vi "Main FPGA 8-axis_2.vi"() -> ()   [LabVIEW 2014]
uses:
  <vilib>/Motion/MotorControl/_s/nism.interpretControlRegister.stateTransition.ctl
  <vilib>/Platform/TimedLoop/XDataNode/timing_clust.ctl
  <vilib>/Platform/TimedLoop/XDataNode/nitl_modes.ctl
  <vilib>/Platform/TimedLoop/XDataNode/wakeup.ctl
  <vilib>/rvi/Emulation/niFpgaGetClockAttributes.vi
  <vilib>/rvi/Emulation/niFpgaSctlEmulationGetInTimedLoop.vi
  <vilib>/rvi/Emulation/niFpgaEmulationReportErrorSimple.vi
  Global FPGA 8-axis.vi
  <vilib>/rvi/eio/common/nirviEmuTemplateMethod_errors.vi
  <vilib>/Motion/MotorControl/_s/nism.interpretControlRegister.indexed.vi
  <vilib>/rvi/Emulation/niFpgaProcessEmulError.vi
  <vilib>/Motion/MotorControl/_s/nism.mdo.read.positionLoopSyncData.vi
  <vilib>/Motion/MotorControl/_s/nism.mdo.read.splineData.vi
  <vilib>/Motion/MotorControl/_s/nism.generateStatusRegister.indexed.vi
  <vilib>/rvi/Emulation/niFpgaCriticalErrorInLSC.vi
  <vilib>/Motion/MotorControl/_s/nism.splineInterpolation.fxp.3.index.vi
  <vilib>/Motion/MotorControl/_s/nism.mdo.handler.indexed.vi
  <vilib>/Motion/SoftMotion/Synchronization/nism.rioScan.generateSyncScan.vi
  <vilib>/eio/EIONode/EIONode.xnode
  <vilib>/Platform/TimedLoop/XDataNode/XDataNode.xnode
  <vilib>/Motion/MotorControl/NI_SoftMotion_MotorControlIP.lvlib
  <vilib>/Platform/TimedLoop/XDataNode/XDNodeRunTimeDep.lvlib
  <vilib>/Motion/SoftMotion/Synchronization/NI_SoftMotion_Synchronization.lvlib
panel:
  in  "Enable Drives?":bool
  out "State":T1=enum."Start --> Initializing" caption="state transition"
  in  "Sync Value":bool
  in  "Sync Enable override?":bool
  in  "Invert direction?":bool
  out "Sync is Fault":bool
  out "Sync is Locked":bool
  in  "minimum pulse":u16=40
  # "Synchronization Loop"
  # "Control Status Loop"
  # "Notes: \n1. This VI provides the communication interface between the NI SoftMotion Engine and the LabVIEW FPGA Module. You must compile this VI for a specific FPGA target before use. After compiling, run the VI before running any of the Express VI examples. For information on moving this example to another FPGA target, refer to ni.com/info and enter info code fpgaex.\n\n2. Only use the Reset Axis button if you are unable to communicate with the axis by any other means. This button resets the device state machine and other VIs to a known state. After resetting the axis, switch the NI Scan Engine from Active Mode to Configuration Mode, then back to Active Mode, before attempting to enable the axis."
  # "(These two buttons \nare for testing\npurposes.)"
  # "Step/Direction Loop"
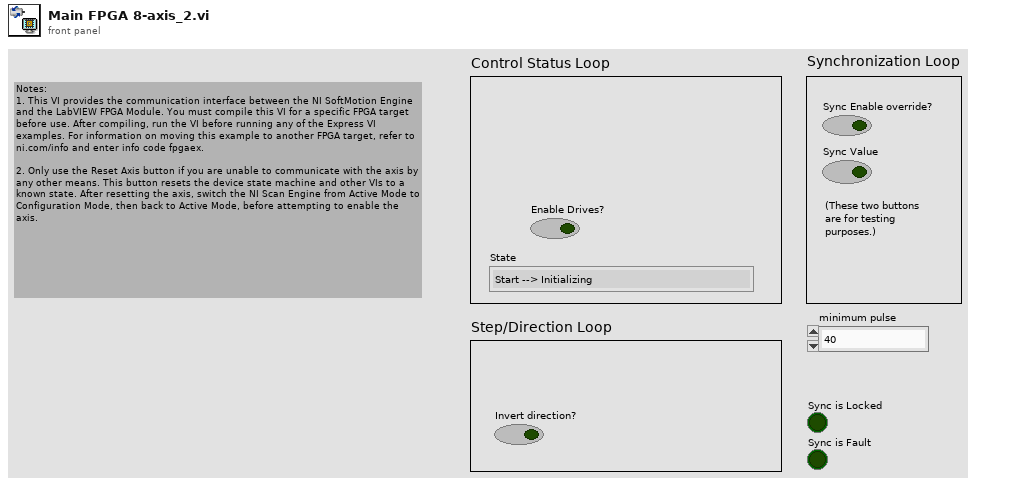
[diagram p1: front panel]
types:
  T1 = typedef "NI_SoftMotion_MotorControlIP.lvlib/nism.interpretControlRegister.stateTransition.ctl" = enum8{"Invalid", "Start --> Initializing", "Initializing --> Disabled", "Disabled --> Ready To Switch On", "Ready To Switch On --> Switched On", "Ready To Switch On --> Disable", "Switched On --> Operation Enable", "Switched On --> Ready To Switch On", "Switched On --> Disabled", "Operation Enable --> Switched On", "Operation Enable --> Ready To Switch On", "Operation Enable --> Disabled", "Fault --> Disabled", "Any --> Fault", "None"}
  T2 = typedef "NI_SoftMotion_MotorControlIP.lvlib/nism.mdo.splineData.ctl" = cluster{"spline type":T3, "traj per/spline per":u16, "spline per/traj per":fxp<+,32,0>}
  T3 = typedef "NI_SoftMotion_MotorControlIP.lvlib/nism.splineInterpolation.type.ctl" = u16
  T4 = typedef "NI_SoftMotion_Synchronization.lvlib/nism.softmotionScan.timerConfig.ctl" = cluster{"target period (clocks)":u16, "host period / target period":u16}
  T5 = typedef "NI_SoftMotion_Synchronization.lvlib/nism.softmotionScan.timerControl.ctl" = cluster{"sm scan":bool, "sm scan count":u32, "sm scan enabled":bool}
  T6 = typedef "XDNodeRunTimeDep.lvlib/timing_clust.ctl" = cluster{"Expected End [f-1]":u64, "Actual End [f-1]":u64, "Finished Late? [f-1]":bool, "Expected End [i-1]":u64, "Actual End [i-1]":u64, "Finished Late? [i-1]":bool, "Expected Start [i]":u64, "Actual Start [i]":u64, "Expected Start [f]":u64, "Actual Start [f]":u64, "Source Name":string, "Structure Name":string, "Period":i64, "Deadline":i64, "Offset":i64, "Start":i64, "Priority":i32, "Timeout":i32, "Mode":T7, "Wakeup Reason":T8, "Error":errorcluster, "Source Type":string, "Secondary Source Type":string, "Global End Time":u64, "Global Start Time":u64, "Frame Duration":u64, "Iteration Duration":u64, "Assigned CPU":i32, "I/O Scan Engine Mode":u32}
  T7 = typedef "XDNodeRunTimeDep.lvlib/nitl_modes.ctl" = enum32{"No Change", "Process missed periods, maintain original phase", "Discard missed periods, maintain original phase", "Process missed periods, ignore original phase", "Discard missed periods, ignore original phase"}
  T8 = typedef "XDNodeRunTimeDep.lvlib/wakeup.ctl" = enum32{"Normal", "Aborted", "Asynchronous wakeup", "Timing source error", "Timed loop error", "Timeout"}
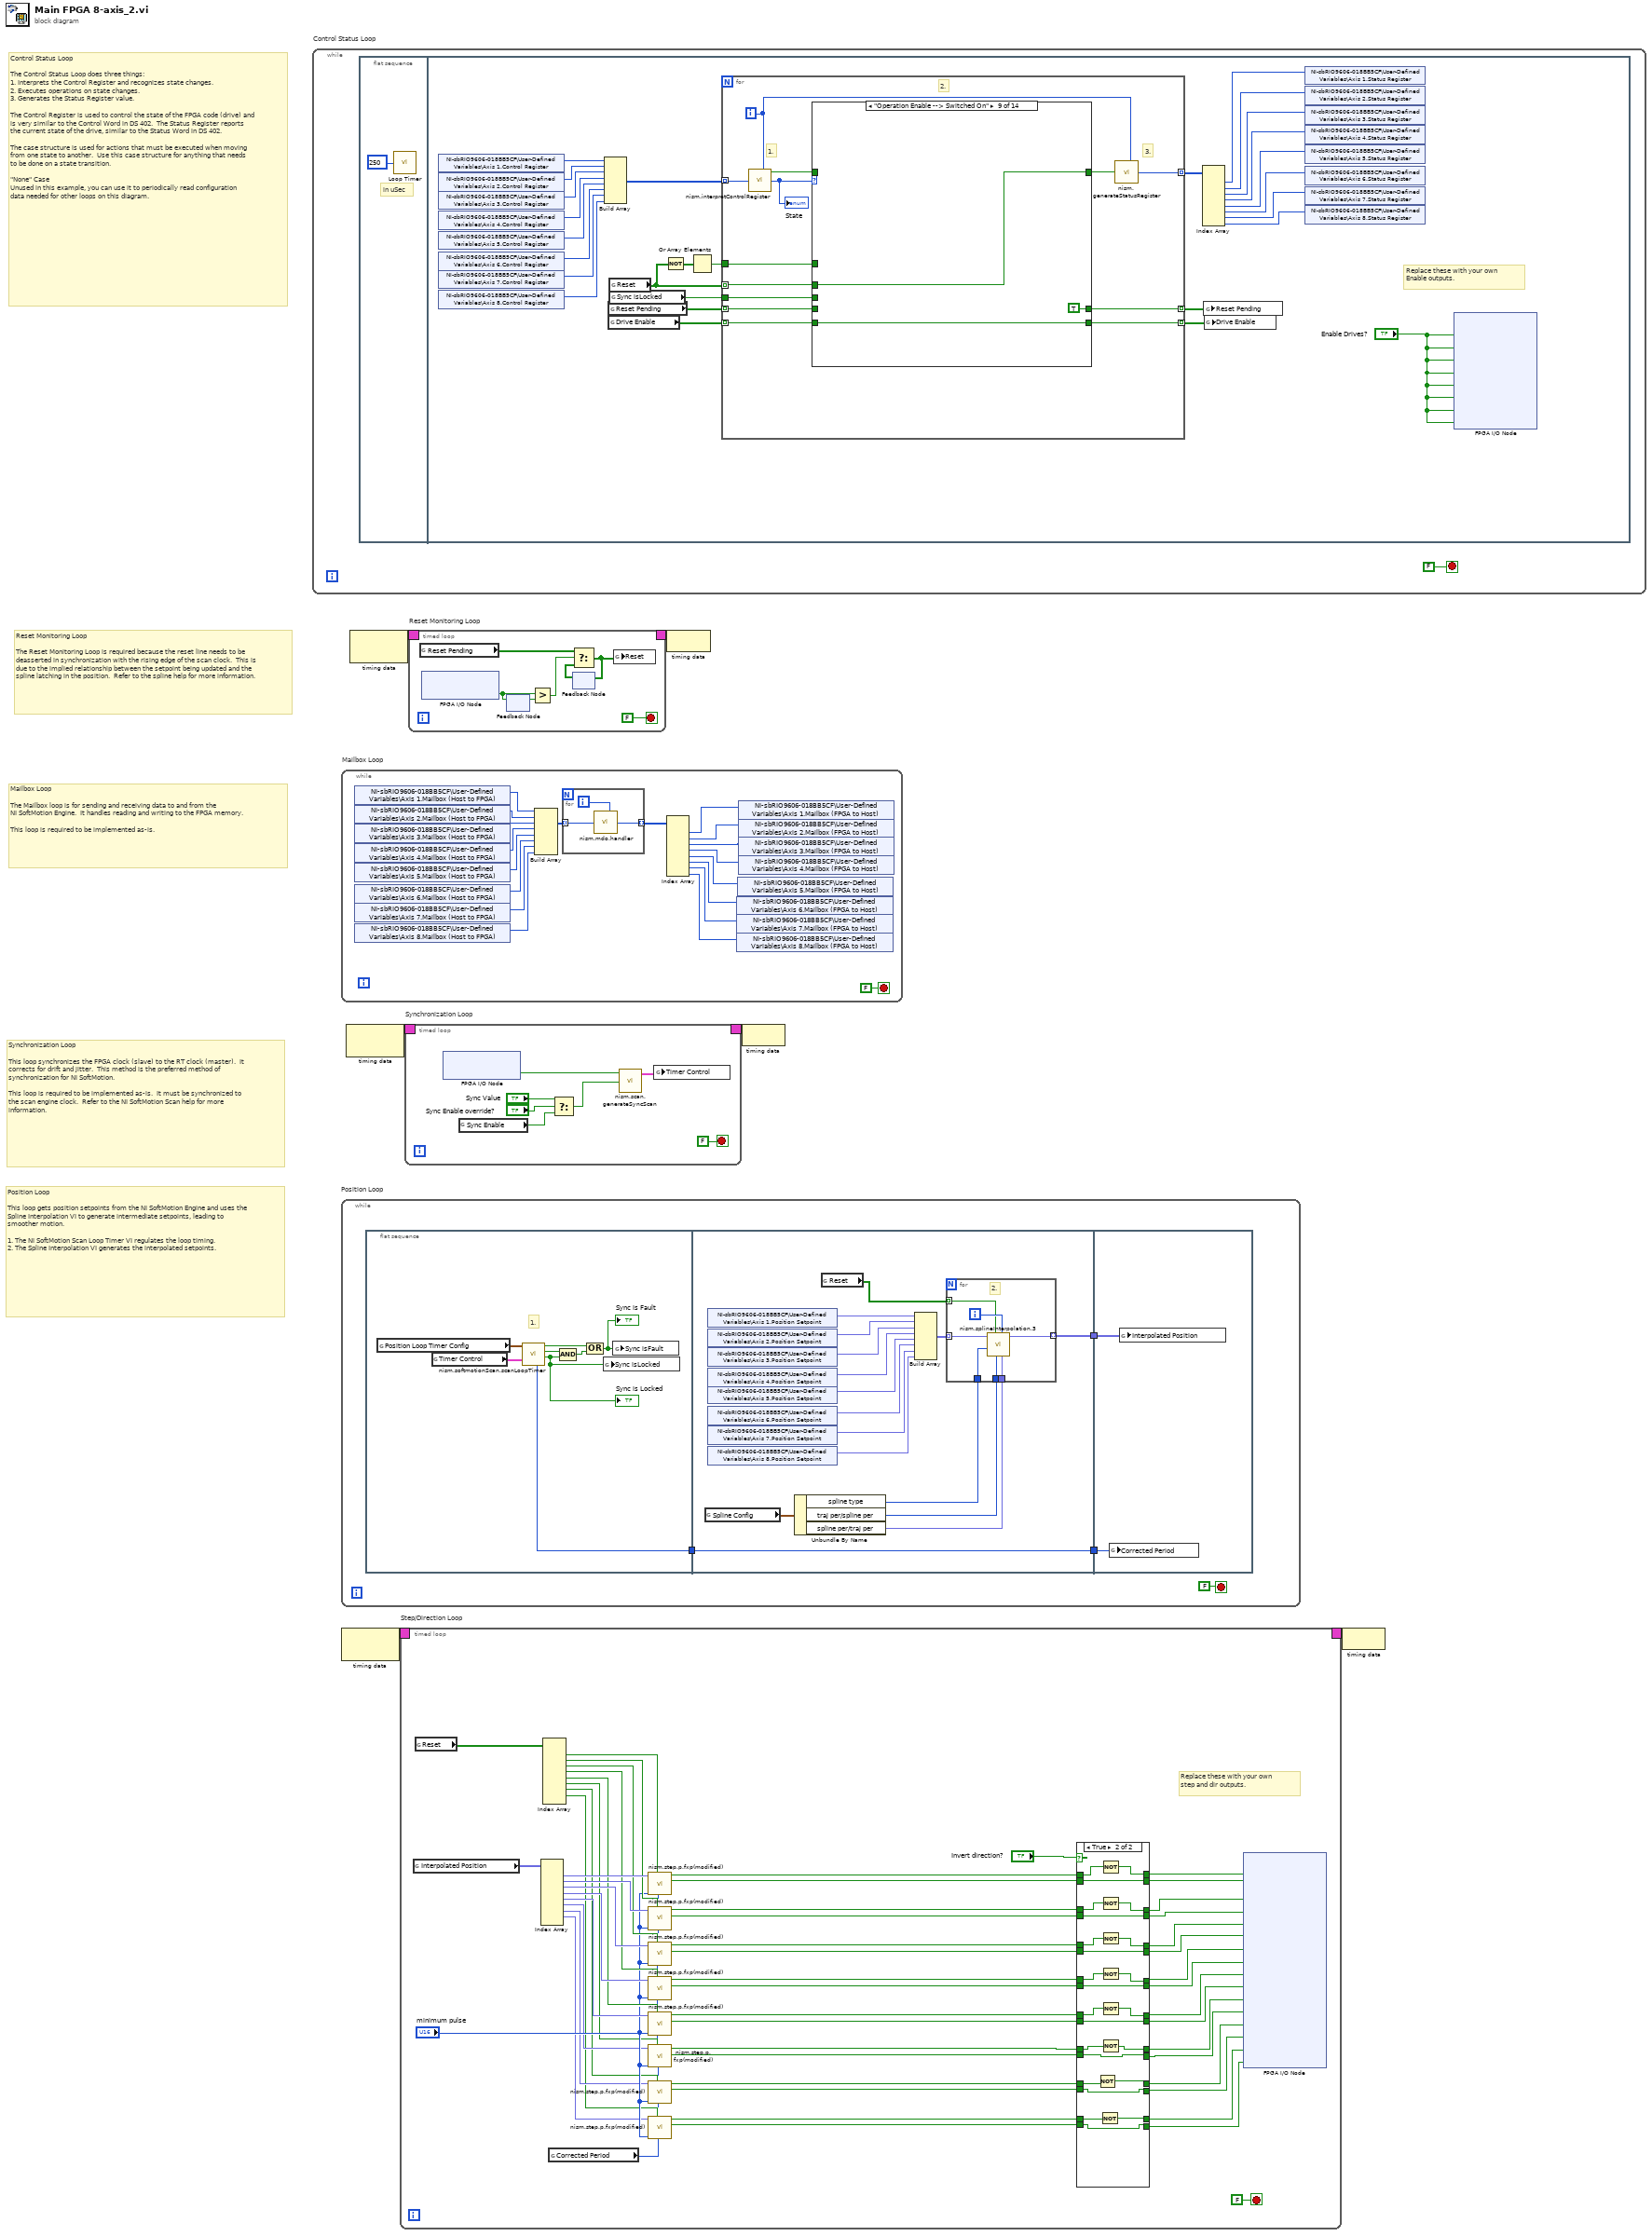
[diagram p0: block diagram]
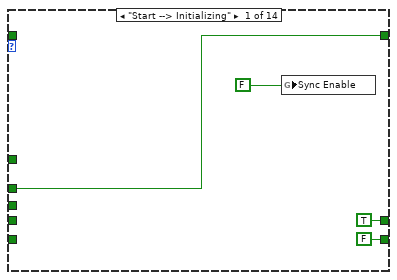
[diagram p3: hidden frame]
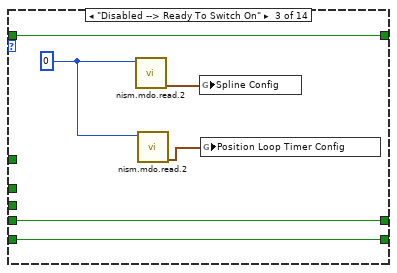
[diagram p5: hidden frame]
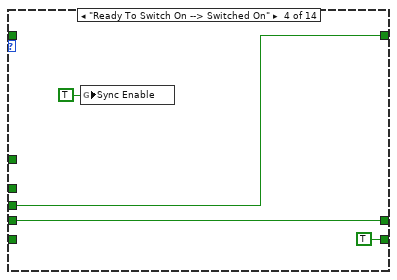
[diagram p6: hidden frame]
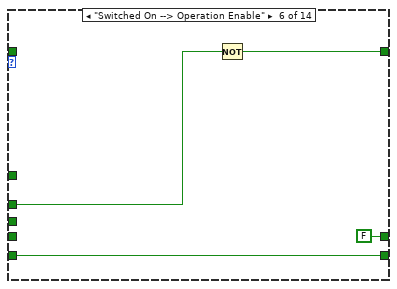
[diagram p8: hidden frame]
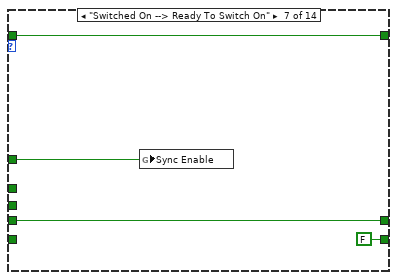
[diagram p9: hidden frame]
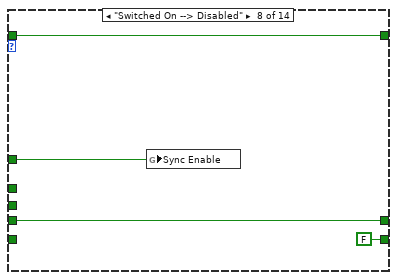
[diagram p10: hidden frame]
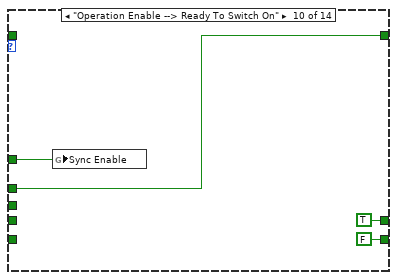
[diagram p11: hidden frame]
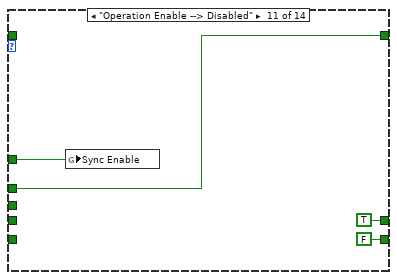
[diagram p12: hidden frame]
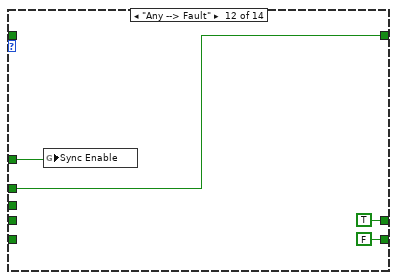
[diagram p13: hidden frame]
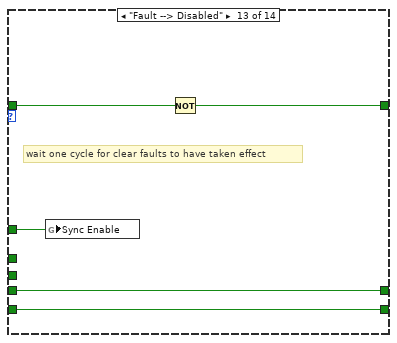
[diagram p14: hidden frame]
diagram:
  # "Position Loop\n\nThis loop gets position setpoints from the NI SoftMotion Engine and uses the Spline Interpolation VI to generate intermediate setpoints, leading to smoother motion.\n\n1. The NI SoftMotion Scan Loop Timer VI regulates the loop timing. \n2. The Spline Interpolation VI generates the interpolated setpoints."
  # "Synchronization Loop\n\nThis loop synchronizes the FPGA clock (slave) to the RT clock (master).  It corrects for drift and jitter.  This method is the preferred method of synchronization for NI SoftMotion.\n\nThis loop is required to be implemented as-is.  It must be synchronized to the scan engine clock.  Refer to the NI SoftMotion Scan help for more information."
  # "Mailbox Loop\n\nThe Mailbox loop is for sending and receiving data to and from the \nNI SoftMotion Engine.  It handles reading and writing to the FPGA memory.\n\nThis loop is required to be implemented as-is."
  # "Reset Monitoring Loop\n\nThe Reset Monitoring Loop is required because the reset line needs to be deasserted in synchronization with the rising edge of the scan clock.  This is due to the implied relationship between the setpoint being updated and the spline latching in the position.  Refer to the spline help for more information."
  # "Control Status Loop\n\nThe Control Status Loop does three things:\n1. Interprets the Control Register and recognizes state changes.\n2. Executes operations on state changes.\n3. Generates the Status Register value.\n\nThe Control Register is used to control the state of the FPGA code (drive) and is very similar to the Control Word in DS 402.  The Status Register reports the current state of the drive, similar to the Status Word in DS 402.\n\nThe case structure is used for actions that must be executed when moving from one state to another.  Use this case structure for anything that needs to be done on a state transition.\n\n\"None\" Case\nUnused in this example, you can use it to periodically read configuration data needed for other loops on this diagram."
  n1 = while "Control Status Loop" {
    stop <- FALSE stop-if-true
    n2 = flat-sequence {
      frame #0 {
        # "in uSec"
        n3 = call "Loop Timer"("Count(uSec)"=u32 250) -> ()  [unwired: 1 out]
      }
      frame #1 {
        # "Replace these with your own\nEnable outputs."
        n4 = shared-variable "NI-sbRIO9606-018BB5CF\\User-Defined Variables\\Axis 1.Control Register"() -> (w25:u32)  [unwired: 1 in, 1 out]
        n5 = shared-variable "NI-sbRIO9606-018BB5CF\\User-Defined Variables\\Axis 2.Control Register"() -> (w24:u32)  [unwired: 1 in, 1 out]
        n6 = shared-variable "NI-sbRIO9606-018BB5CF\\User-Defined Variables\\Axis 3.Control Register"() -> (w23:u32)  [unwired: 1 in, 1 out]
        n7 = shared-variable "NI-sbRIO9606-018BB5CF\\User-Defined Variables\\Axis 4.Control Register"() -> (w22:u32)  [unwired: 1 in, 1 out]
        n8 = shared-variable "NI-sbRIO9606-018BB5CF\\User-Defined Variables\\Axis 5.Control Register"() -> (w21:u32)  [unwired: 1 in, 1 out]
        n9 = shared-variable "NI-sbRIO9606-018BB5CF\\User-Defined Variables\\Axis 6.Control Register"() -> (w15:u32)  [unwired: 1 in, 1 out]
        n10 = shared-variable "NI-sbRIO9606-018BB5CF\\User-Defined Variables\\Axis 7.Control Register"() -> (w14:u32)  [unwired: 1 in, 1 out]
        n11 = shared-variable "NI-sbRIO9606-018BB5CF\\User-Defined Variables\\Axis 8.Control Register"() -> (w13:u32)  [unwired: 1 in, 1 out]
        n12 = Build Array(w25, w24, w23, w22, w21, w15, w14, w13) -> (w34:u32[])
        n13 = global read "Global FPGA 8-axis.vi" "Reset Pending"() -> (w29:bool[])
        n14 = global read "Global FPGA 8-axis.vi" "Drive Enable"() -> (w28:bool[])
        n15 = global read "Global FPGA 8-axis.vi" "Reset"() -> (w30:bool[])
        n16 = global read "Global FPGA 8-axis.vi" "Sync isLocked"() -> (w35:bool)
        n17 = Not(x=w30) -> (.not. x?=w32:bool[])
        n18 = Or Array Elements(Boolean array=w32) -> (logical OR=w31:bool)
        n19 = for {
          tunnel: w30 -> [w43] mode=indexing
          tunnel: w35 -> [w42]
          tunnel: w34 -> [w44] mode=indexing
          tunnel: [w41] -> w26 mode=indexing
          tunnel: [w40] -> w33 mode=indexing
          tunnel: [w39] -> w27 mode=indexing
          tunnel: w31 -> [w38]
          tunnel: w29 -> [w37] mode=indexing
          tunnel: w28 -> [w36] mode=indexing
          i -> [w45]
          # "3."
          # "2."
          # "1."
          n20 = call-poly <vilib>:"nism.interpretControlRegister.vi"("control register"=w44, "axis index"=w45) -> ("transition occurred"=w46:bool, "state transition"=w47:T1)  [unwired: 6 in]
          "State" <- w47
          n21 = case shown="\"Operation Enable --> Switched On\"" w47 {
            tunnel: w46 -> [_ w55 w61 _ w68 _ w76 w80 _ _ _ _ w100 _]
            tunnel: [w52 w55 w61 w63 w68 w72 w76 w80 w82 w85 w89 w93 w99 _] -> w48
            tunnel: w43 -> [w52 _ _ _ _ w71 _ _ w82 w85 w89 w93 _ _]
            tunnel: w42 -> [_ _ _ w63 _ _ _ _ _ _ _ _ _ _]
            tunnel: [TRUE ("Write.Reset Pending") w54 w57 w62 w67 FALSE ("Write.Reset Pending") w73 w77 TRUE ("Write.Reset Pending") TRUE ("Write.Reset Pending") TRUE ("Write.Reset Pending") TRUE ("Write.Reset Pending") w97 w102] -> w40
            tunnel: [FALSE ("Write.Drive Enable") w53 w56 TRUE ("Write.Drive Enable") w66 w69 FALSE ("Write.Drive Enable") FALSE ("Write.Drive Enable") w81 FALSE ("Write.Drive Enable") FALSE ("Write.Drive Enable") FALSE ("Write.Drive Enable") w96 w101] -> w39
            tunnel: w38 -> [_ _ _ _ _ _ w74 w78 _ w84 w88 w92 w98 _]
            tunnel: w37 -> [_ w54 w57 w62 w67 _ w73 w77 _ _ _ _ w97 w102]
            tunnel: w36 -> [_ w53 w56 _ w66 w69 _ _ w81 _ _ _ w96 w101]
            frame "Start --> Initializing" {
              n22 = global write "Global FPGA 8-axis.vi" "Sync Enable"(FALSE ("Sync Enable")) -> ()
            }
            frame "Initializing --> Disabled" {
            }
            frame "Disabled --> Ready To Switch On" {
              w59 = 0 ("axis index")
              n23 = call-poly <vilib>:"nism.mdo.read.2.vi"("axis index"=w59) -> ("spline"=w60:T2)  [unwired: 10 in]
              n24 = call-poly <vilib>:"nism.mdo.read.2.vi"("axis index"=w59) -> ("position loop sync"=w58:T4)  [unwired: 10 in]
              n25 = global write "Global FPGA 8-axis.vi" "Spline Config"(w60) -> ()
              n26 = global write "Global FPGA 8-axis.vi" "Position Loop Timer Config"(w58) -> ()
            }
            frame "Ready To Switch On --> Switched On" {
              n27 = global write "Global FPGA 8-axis.vi" "Sync Enable"(TRUE ("Sync Enable")) -> ()
            }
            frame "Ready To Switch On --> Disable" {
            }
            frame "Switched On --> Operation Enable" {
              n28 = Not(x=w71) -> (.not. x?=w72:bool)
            }
            frame "Switched On --> Ready To Switch On" {
              n29 = global write "Global FPGA 8-axis.vi" "Sync Enable"(w74) -> ()
            }
            frame "Switched On --> Disabled" {
              n30 = global write "Global FPGA 8-axis.vi" "Sync Enable"(w78) -> ()
            }
            frame "Operation Enable --> Switched On" {
            }
            frame "Operation Enable --> Ready To Switch On" {
              n31 = global write "Global FPGA 8-axis.vi" "Sync Enable"(w84) -> ()
            }
            frame "Operation Enable --> Disabled" {
              n32 = global write "Global FPGA 8-axis.vi" "Sync Enable"(w88) -> ()
            }
            frame "Any --> Fault" {
              n33 = global write "Global FPGA 8-axis.vi" "Sync Enable"(w92) -> ()
            }
            frame "Fault --> Disabled" {
              # "wait one cycle for clear faults to have taken effect"
              n34 = global write "Global FPGA 8-axis.vi" "Sync Enable"(w98) -> ()
              n35 = Not(x=w100) -> (.not. x?=w99:bool)
            }
            frame "None", Default {
            }
          }
          n36 = call-poly <vilib>:"nism.generateStatusRegister.vi"("transition success"=w48, "axis index"=w45) -> ("status register"=w41:u32)  [unwired: 7 in]
        }
        n37 = Index Array(array=w26) -> (element #1=w20:u32, element #2=w19:u32, element #3=w18:u32, element #4=w17:u32, element #5=w16:u32, element #6=w12:u32, element #7=w11:u32, element #8=w10:u32)  [unwired: 8 in]
        n38 = global write "Global FPGA 8-axis.vi" "Reset Pending"(w33) -> ()
        n39 = global write "Global FPGA 8-axis.vi" "Drive Enable"(w27) -> ()
        n40 = shared-variable "NI-sbRIO9606-018BB5CF\\User-Defined Variables\\Axis 1.Status Register"(w20) -> ()  [unwired: 1 in, 1 out]
        n41 = shared-variable "NI-sbRIO9606-018BB5CF\\User-Defined Variables\\Axis 2.Status Register"(w19) -> ()  [unwired: 1 in, 1 out]
        n42 = shared-variable "NI-sbRIO9606-018BB5CF\\User-Defined Variables\\Axis 3.Status Register"(w18) -> ()  [unwired: 1 in, 1 out]
        n43 = shared-variable "NI-sbRIO9606-018BB5CF\\User-Defined Variables\\Axis 4.Status Register"(w17) -> ()  [unwired: 1 in, 1 out]
        n44 = shared-variable "NI-sbRIO9606-018BB5CF\\User-Defined Variables\\Axis 5.Status Register"(w16) -> ()  [unwired: 1 in, 1 out]
        n45 = shared-variable "NI-sbRIO9606-018BB5CF\\User-Defined Variables\\Axis 6.Status Register"(w12) -> ()  [unwired: 1 in, 1 out]
        n46 = shared-variable "NI-sbRIO9606-018BB5CF\\User-Defined Variables\\Axis 7.Status Register"(w11) -> ()  [unwired: 1 in, 1 out]
        n47 = shared-variable "NI-sbRIO9606-018BB5CF\\User-Defined Variables\\Axis 8.Status Register"(w10) -> ()  [unwired: 1 in, 1 out]
        n48 = xnode "FPGA I/O Node"("RMC/DIO15"="Enable Drives?", "RMC/DIO79"="Enable Drives?", "RMC/DIO78"="Enable Drives?", "RMC/DIO13"="Enable Drives?", "RMC/DIO62"="Enable Drives?", "RMC/DIO61"="Enable Drives?", "RMC/DIO76"="Enable Drives?", "RMC/DIO11"="Enable Drives?") -> ()  [unwired: 8 in, 8 out]
      }
    }
  }
  n49 = while "Position Loop" {
    stop <- FALSE stop-if-true
    n50 = flat-sequence {
      tunnel: [w107] -> w103
      tunnel: [w124] -> w105
      tunnel: [w123] -> w104
      tunnel: w103 -> [w123]
      tunnel: w105 -> [w138]
      tunnel: w104 -> [w139]
      frame #0 {
        # "1."
        n51 = global read "Global FPGA 8-axis.vi" "Position Loop Timer Config"() -> (w109:T4)
        n52 = global read "Global FPGA 8-axis.vi" "Timer Control"() -> (w108:T5)
        n53 = call <vilib>:"nism.softmotionScan.scanLoopTimer.vi"("timer control"=w108, "timer config"=w109) -> ("scan running?"=w111:bool, "finished late?"=w113:bool, "fault occurred?"=w114:bool, "corrected period"=w107:u16)  [unwired: 5 in, 1 out]
        "Sync is Locked" <- w111
        n54 = Compound Arithmetic op=AND(w113, w111) -> (w112:bool)
        n55 = Compound Arithmetic op=OR(w114, w112) -> (w110:bool)
        "Sync is Fault" <- w110
        n56 = global write "Global FPGA 8-axis.vi" "Sync isLocked"(w111) -> ()
        n57 = global write "Global FPGA 8-axis.vi" "Sync isFault"(w110) -> ()
      }
      frame #1 {
        n58 = global read "Global FPGA 8-axis.vi" "Spline Config"() -> (w126:T2)
        n59 = shared-variable "NI-sbRIO9606-018BB5CF\\User-Defined Variables\\Axis 1.Position Setpoint"() -> (w122:fxp<+/-,64,32>)  [unwired: 1 in, 1 out]
        n60 = shared-variable "NI-sbRIO9606-018BB5CF\\User-Defined Variables\\Axis 2.Position Setpoint"() -> (w121:fxp<+/-,64,32>)  [unwired: 1 in, 1 out]
        n61 = shared-variable "NI-sbRIO9606-018BB5CF\\User-Defined Variables\\Axis 3.Position Setpoint"() -> (w120:fxp<+/-,64,32>)  [unwired: 1 in, 1 out]
        n62 = shared-variable "NI-sbRIO9606-018BB5CF\\User-Defined Variables\\Axis 4.Position Setpoint"() -> (w119:fxp<+/-,64,32>)  [unwired: 1 in, 1 out]
        n63 = shared-variable "NI-sbRIO9606-018BB5CF\\User-Defined Variables\\Axis 5.Position Setpoint"() -> (w118:fxp<+/-,64,32>)  [unwired: 1 in, 1 out]
        n64 = shared-variable "NI-sbRIO9606-018BB5CF\\User-Defined Variables\\Axis 6.Position Setpoint"() -> (w117:fxp<+/-,64,32>)  [unwired: 1 in, 1 out]
        n65 = shared-variable "NI-sbRIO9606-018BB5CF\\User-Defined Variables\\Axis 7.Position Setpoint"() -> (w116:fxp<+/-,64,32>)  [unwired: 1 in, 1 out]
        n66 = shared-variable "NI-sbRIO9606-018BB5CF\\User-Defined Variables\\Axis 8.Position Setpoint"() -> (w115:fxp<+/-,64,32>)  [unwired: 1 in, 1 out]
        n67 = Unbundle By Name(w126) -> ("spline type"=w130:T3, "traj per/spline per"=w129:u16, "spline per/traj per"=w128:fxp<+,32,0>)
        n68 = global read "Global FPGA 8-axis.vi" "Reset"() -> (w125:bool[])
        n69 = Build Array(w122, w121, w120, w119, w118, w117, w116, w115) -> (w127:fxp<+/-,64,32>[])
        n70 = for {
          tunnel: w130 -> [w137]
          tunnel: w129 -> [w136]
          tunnel: w128 -> [w135]
          tunnel: w125 -> [w132] mode=indexing
          tunnel: w127 -> [w134] mode=indexing
          tunnel: [w131] -> w124 mode=indexing
          i -> [w133]
          # "2."
          n71 = call-poly <vilib>:"nism.splineInterpolation.3.vi"("1 / calls per sample"=w135, "index"=w133, "calls per sample"=w136, "reset"=w132, "spline type"=w137, "x"=w134) -> ("xi"=w131:fxp<+/-,64,32>)  [unwired: 4 in, 1 out]
        }
      }
      frame #2 {
        n72 = global write "Global FPGA 8-axis.vi" "Corrected Period"(w139) -> ()
        n73 = global write "Global FPGA 8-axis.vi" "Interpolated Position"(w138) -> ()
      }
    }
  }
  n74 = node-c288() -> (w6:T6)  [unwired: 1 in]
  n75 = while "Mailbox Loop" {
    stop <- FALSE stop-if-true
    n76 = shared-variable "NI-sbRIO9606-018BB5CF\\User-Defined Variables\\Axis 1.Mailbox (Host to FPGA)"() -> (w155:u64)  [unwired: 1 in, 1 out]
    n77 = shared-variable "NI-sbRIO9606-018BB5CF\\User-Defined Variables\\Axis 2.Mailbox (Host to FPGA)"() -> (w154:u64)  [unwired: 1 in, 1 out]
    n78 = shared-variable "NI-sbRIO9606-018BB5CF\\User-Defined Variables\\Axis 3.Mailbox (Host to FPGA)"() -> (w153:u64)  [unwired: 1 in, 1 out]
    n79 = shared-variable "NI-sbRIO9606-018BB5CF\\User-Defined Variables\\Axis 4.Mailbox (Host to FPGA)"() -> (w152:u64)  [unwired: 1 in, 1 out]
    n80 = shared-variable "NI-sbRIO9606-018BB5CF\\User-Defined Variables\\Axis 5.Mailbox (Host to FPGA)"() -> (w151:u64)  [unwired: 1 in, 1 out]
    n81 = shared-variable "NI-sbRIO9606-018BB5CF\\User-Defined Variables\\Axis 6.Mailbox (Host to FPGA)"() -> (w145:u64)  [unwired: 1 in, 1 out]
    n82 = shared-variable "NI-sbRIO9606-018BB5CF\\User-Defined Variables\\Axis 7.Mailbox (Host to FPGA)"() -> (w144:u64)  [unwired: 1 in, 1 out]
    n83 = shared-variable "NI-sbRIO9606-018BB5CF\\User-Defined Variables\\Axis 8.Mailbox (Host to FPGA)"() -> (w143:u64)  [unwired: 1 in, 1 out]
    n84 = Build Array(w155, w154, w153, w152, w151, w145, w144, w143) -> (w157:u64[])
    n85 = for {
      tunnel: w157 -> [w161] mode=indexing
      tunnel: [w160] -> w156 mode=indexing
      i -> [w159]
      n86 = call-poly <vilib>:"nism.mdo.handler.vi"("mbox (host to fpga)"=w161, "axis index"=w159) -> ("mbox (fpga to host)"=w160:u64)  [unwired: 7 in]
    }
    n87 = Index Array(array=w156) -> (element #1=w150:u64, element #2=w149:u64, element #3=w148:u64, element #4=w147:u64, element #5=w146:u64, element #6=w142:u64, element #7=w141:u64, element #8=w140:u64)  [unwired: 8 in]
    n88 = shared-variable "NI-sbRIO9606-018BB5CF\\User-Defined Variables\\Axis 6.Mailbox (FPGA to Host)"(w142) -> ()  [unwired: 1 in, 1 out]
    n89 = shared-variable "NI-sbRIO9606-018BB5CF\\User-Defined Variables\\Axis 7.Mailbox (FPGA to Host)"(w141) -> ()  [unwired: 1 in, 1 out]
    n90 = shared-variable "NI-sbRIO9606-018BB5CF\\User-Defined Variables\\Axis 8.Mailbox (FPGA to Host)"(w140) -> ()  [unwired: 1 in, 1 out]
    n91 = shared-variable "NI-sbRIO9606-018BB5CF\\User-Defined Variables\\Axis 5.Mailbox (FPGA to Host)"(w146) -> ()  [unwired: 1 in, 1 out]
    n92 = shared-variable "NI-sbRIO9606-018BB5CF\\User-Defined Variables\\Axis 1.Mailbox (FPGA to Host)"(w150) -> ()  [unwired: 1 in, 1 out]
    n93 = shared-variable "NI-sbRIO9606-018BB5CF\\User-Defined Variables\\Axis 2.Mailbox (FPGA to Host)"(w149) -> ()  [unwired: 1 in, 1 out]
    n94 = shared-variable "NI-sbRIO9606-018BB5CF\\User-Defined Variables\\Axis 3.Mailbox (FPGA to Host)"(w148) -> ()  [unwired: 1 in, 1 out]
    n95 = shared-variable "NI-sbRIO9606-018BB5CF\\User-Defined Variables\\Axis 4.Mailbox (FPGA to Host)"(w147) -> ()  [unwired: 1 in, 1 out]
  }
  n96 = node-c288() -> (w4:T6)  [unwired: 1 in]
  n97 = node-c288() -> (w2:T6)  [unwired: 1 in]
  n98 = timed-loop "Step/Direction Loop" {
    timing: w6 -> [_]
    timing-out: [_] -> w5
    stop <- FALSE stop-if-true
    # "Replace these with your own\nstep and dir outputs."
    n99 = global read "Global FPGA 8-axis.vi" "Interpolated Position"() -> (w214:fxp<+/-,64,32>[])
    n100 = global read "Global FPGA 8-axis.vi" "Reset"() -> (w208:bool[])
    n101 = Index Array(array=w214) -> (element #1=w213:fxp<+/-,64,32>, element #2=w212:fxp<+/-,64,32>, element #3=w211:fxp<+/-,64,32>, element #4=w210:fxp<+/-,64,32>, element #5=w209:fxp<+/-,64,32>, element #6=w184:fxp<+/-,64,32>, element #7=w183:fxp<+/-,64,32>, element #8=w182:fxp<+/-,64,32>)  [unwired: 9 in, 1 out]
    n102 = Index Array(array=w208) -> (element #1=w207:bool, element #2=w206:bool, element #3=w205:bool, element #4=w204:bool, element #5=w203:bool, element #6=w181:bool, element #7=w180:bool, element #8=w179:bool)  [unwired: 9 in, 1 out]
    n103 = global read "Global FPGA 8-axis.vi" "Corrected Period"() -> (w172:u16)
    n104 = call "nism.step.p.fxp(modified).vi"("calls per sample"=w172, "reset"=w207, "minimum pulse"="minimum pulse", "position setpoint"=w213) -> ("step"=w201:bool, "direction"=w202:bool)  [unwired: 4 in, 2 out]
    n105 = call "nism.step.p.fxp(modified).vi"("calls per sample"=w172, "reset"=w206, "minimum pulse"="minimum pulse", "position setpoint"=w212) -> ("step"=w199:bool, "direction"=w200:bool)  [unwired: 4 in, 2 out]
    n106 = call "nism.step.p.fxp(modified).vi"("calls per sample"=w172, "reset"=w205, "minimum pulse"="minimum pulse", "position setpoint"=w211) -> ("step"=w197:bool, "direction"=w198:bool)  [unwired: 4 in, 2 out]
    n107 = call "nism.step.p.fxp(modified).vi"("calls per sample"=w172, "reset"=w204, "minimum pulse"="minimum pulse", "position setpoint"=w210) -> ("step"=w195:bool, "direction"=w196:bool)  [unwired: 4 in, 2 out]
    n108 = call "nism.step.p.fxp(modified).vi"("calls per sample"=w172, "reset"=w203, "minimum pulse"="minimum pulse", "position setpoint"=w209) -> ("step"=w193:bool, "direction"=w194:bool)  [unwired: 4 in, 2 out]
    n109 = call "nism.step.p.fxp(modified).vi"("calls per sample"=w172, "reset"=w181, "minimum pulse"="minimum pulse", "position setpoint"=w184) -> ("step"=w190:bool, "direction"=w191:bool)  [unwired: 4 in, 2 out]
    n110 = call "nism.step.p.fxp(modified).vi"("calls per sample"=w172, "reset"=w180, "minimum pulse"="minimum pulse", "position setpoint"=w183) -> ("step"=w188:bool, "direction"=w189:bool)  [unwired: 4 in, 2 out]
    n111 = call "nism.step.p.fxp(modified).vi"("calls per sample"=w172, "reset"=w179, "minimum pulse"="minimum pulse", "position setpoint"=w182) -> ("step"=w186:bool, "direction"=w187:bool)  [unwired: 4 in, 2 out]
    n112 = case shown="True" "Invert direction?" {
      tunnel: w202 -> [w231 w255]
      tunnel: [w231 w254] -> w171
      tunnel: w200 -> [w229 w253]
      tunnel: [w229 w252] -> w169
      tunnel: w198 -> [w227 w251]
      tunnel: [w227 w250] -> w167
      tunnel: w196 -> [w225 w249]
      tunnel: [w225 w248] -> w165
      tunnel: w194 -> [w223 w247]
      tunnel: [w223 w246] -> w163
      tunnel: w201 -> [w230 w245]
      tunnel: [w230 w245] -> w170
      tunnel: w199 -> [w228 w244]
      tunnel: [w228 w244] -> w168
      tunnel: w197 -> [w226 w243]
      tunnel: [w226 w243] -> w166
      tunnel: w195 -> [w224 w242]
      tunnel: [w224 w242] -> w164
      tunnel: w193 -> [w222 w241]
      tunnel: [w222 w241] -> w162
      tunnel: w191 -> [w221 w240]
      tunnel: w190 -> [w220 w233]
      tunnel: w189 -> [w219 w239]
      tunnel: w188 -> [w218 w235]
      tunnel: w187 -> [w217 w238]
      tunnel: w186 -> [w216 w236]
      tunnel: [w221 w232] -> w178
      tunnel: [w220 w233] -> w177
      tunnel: [w219 w234] -> w176
      tunnel: [w218 w235] -> w175
      tunnel: [w217 w237] -> w174
      tunnel: [w216 w236] -> w173
      frame False {
      }
      frame True {
        n113 = Not(x=w239) -> (.not. x?=w234:bool)
        n114 = Not(x=w238) -> (.not. x?=w237:bool)
        n115 = Not(x=w255) -> (.not. x?=w254:bool)
        n116 = Not(x=w253) -> (.not. x?=w252:bool)
        n117 = Not(x=w251) -> (.not. x?=w250:bool)
        n118 = Not(x=w249) -> (.not. x?=w248:bool)
        n119 = Not(x=w247) -> (.not. x?=w246:bool)
        n120 = Not(x=w240) -> (.not. x?=w232:bool)
      }
    }
    n121 = xnode "FPGA I/O Node"("RMC/DIO46"=w171, "RMC/DIO47"=w170, "RMC/DIO14"=w169, "RMC/DIO63"=w168, "RMC/DIO95"=w167, "RMC/DIO31"=w166, "RMC/DIO30"=w165, "RMC/DIO45"=w164, "RMC/DIO77"=w163, "RMC/DIO44"=w162, "RMC/DIO12"=w178, "RMC/DIO94"=w177, "RMC/DIO93"=w176, "RMC/DIO29"=w175, "RMC/DIO28"=w174, "RMC/DIO43"=w173) -> ()  [unwired: 16 in, 16 out]
  }
  n122 = timed-loop "Synchronization Loop" {
    timing: w4 -> [_]
    timing-out: [_] -> w3
    stop <- FALSE stop-if-true
    n123 = xnode "FPGA I/O Node"() -> ("Scan Clock"=w262:bool)  [unwired: 1 in, 1 out]
    n124 = global read "Global FPGA 8-axis.vi" "Sync Enable"() -> (w261:bool)
    n125 = Select(t="Sync Value", s="Sync Enable override?", f=w261) -> (s? t:f=w258:bool)
    n126 = call-poly <vilib>:"nism.scan.generateSyncScan.vi"("scan enable?"=w258, "scan clock"=w262) -> ("timer control"=w263:T5)  [unwired: 3 in]
    n127 = global write "Global FPGA 8-axis.vi" "Timer Control"(w263) -> ()
  }
  n128 = timed-loop "Reset Monitoring Loop" {
    timing: w2 -> [_]
    timing-out: [_] -> w1
    stop <- FALSE stop-if-true
    n129 = global read "Global FPGA 8-axis.vi" "Reset Pending"() -> (w269:bool[])
    n130 = xnode "FPGA I/O Node"() -> ("Scan Clock"=w268:bool)  [unwired: 1 in, 1 out]
    n131 = feedback-in #1(w268) -> ()
    n132 = feedback #1() -> (w267:bool)  [unwired: 1 in]
    n133 = Greater?(x=w268, y=w267) -> (0:w273:bool)
    n134 = feedback #2() -> (w272:bool[])  [unwired: 1 in]
    n135 = Select(t=w269, s=w273, f=w272) -> (s? t:f=w270:bool[])
    n136 = feedback-in #2(w270) -> ()
    n137 = global write "Global FPGA 8-axis.vi" "Reset"(w270) -> ()
  }
  n138 = node-c288(w1) -> ()
  n139 = node-c288(w3) -> ()
  n140 = node-c288(w5) -> ()
